vi "X Axis Format String Write.vi"(8 "error in (no error)":errorcluster, 9 "X Axis Format":string, 11 "3D Plot.lvclass in":refnum<class "3D Plot.lvclass">) -> (0 "error out":errorcluster, 3 "3D Plot.lvclass out":refnum<class "3D Plot.lvclass">)   [LabVIEW 2020, in "3D Plot.lvclass"]
uses:
  3D Plot.lvclass
  3D Plot.lvclass/3D Plot.ctl
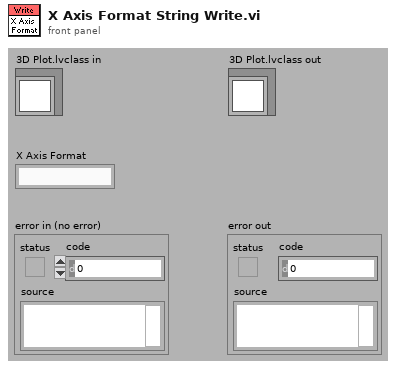
[diagram p1: front panel]
types:
  T1 = typedef "3D Plot.lvclass/Format Property.ctl" = string[]
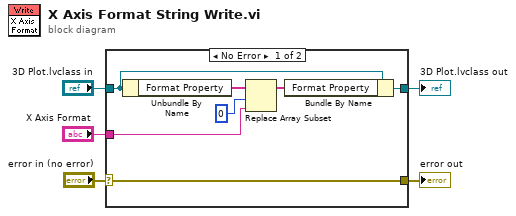
[diagram p0: block diagram]
diagram:
  n1 = case shown="No Error" "error in (no error)" {
    selector: "error in (no error)" -> [w12 w13]
    tunnel: "X Axis Format" -> [w10 _]
    tunnel: "3D Plot.lvclass in" -> [w7 w14]
    tunnel: [w6 w14] -> w3
    tunnel: [w12 w13] -> w1
    frame No Error {
      n2 = Unbundle By Name(w7) -> ("Format Property"=w11:T1)
      n3 = Replace Array Subset(array=w11, new element=w10, index=0) -> (w8:T1)
      n4 = Bundle By Name(cluster=w7, "Format Property"=w8) -> (w6:refnum<class "3D Plot.lvclass">)
    }
    frame Error {
    }
  }
  "3D Plot.lvclass out" <- w3
  "error out" <- w1
